vi "Test Assert Not Error.vi"(8 "error in (no error)":errorcluster) -> (0 "error out":errorcluster)   [LabVIEW 2009]
uses:
  classes/Assert/Assert.lvclass
  classes/Test/Test.lvclass
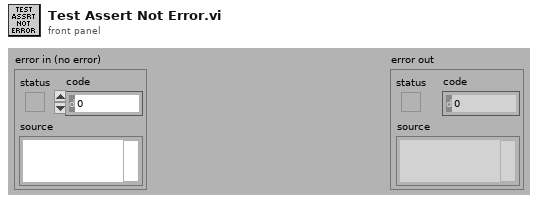
[diagram p1: front panel]
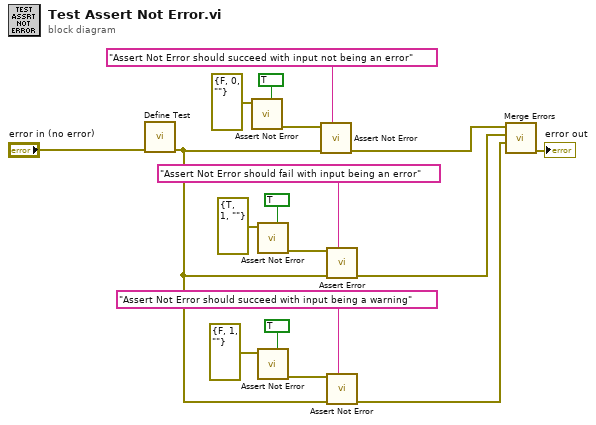
[diagram p0: block diagram]
diagram:
  n1 = call "Define Test.vi"("error in (no error)"="error in (no error)") -> ("error out"=w3:errorcluster)  [unwired: 10 in]
  n2 = call "Assert Not Error.vi"("Assert Only? (F)"=TRUE, "Not Error?"=errorcluster {"status"=FALSE, "code"=0, "source"=""} ("Error?")) -> ("error out"=w18:errorcluster)  [unwired: 9 in]
  n3 = call "Assert Not Error.vi"("Assert Only? (F)"=TRUE, "Not Error?"=errorcluster {"status"=TRUE, "code"=1, "source"=""} ("Error?")) -> ("error out"=w16:errorcluster)  [unwired: 9 in]
  n4 = call "Assert Not Error.vi"("Assert Only? (F)"=TRUE, "Not Error?"=errorcluster {"status"=FALSE, "code"=1, "source"=""} ("Error?")) -> ("error out"=w6:errorcluster)  [unwired: 9 in]
  n5 = call "Assert Not Error.vi"("Label"="Assert Not Error should succeed with input not being an error", "error in (no error)"=w3, "Not Error?"=w18) -> ("error out"=w10:errorcluster)  [unwired: 8 in]
  n6 = call "Assert Error.vi"("Label"="Assert Not Error should fail with input being an error", "error in (no error)"=w3, "Error?"=w16) -> ("error out"=w11:errorcluster)  [unwired: 8 in]
  n7 = call "Assert Not Error.vi"("Label"="Assert Not Error should succeed with input being a warning", "error in (no error)"=w3, "Not Error?"=w6) -> ("error out"=w1:errorcluster)  [unwired: 8 in]
  n8 = call <vilib>:"Merge Errors.vi"("error in 3 (no error)"=w1, "error in 2 (no error)"=w11, "error in 1 (no error)"=w10) -> ("error out"=→"error out":errorcluster)  [unwired: 4 in]
